vi "ErrorOut.vi"(1 "error in":errorcluster, 2 "DNL_NodeType":T1(ring)) -> (0 "error out":errorcluster)   [LabVIEW 2020]
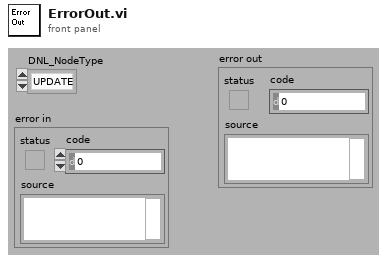
[diagram p1: front panel]
types:
  T1 = enum16{"UPDATE", "READ", "QUERY", "CREATE CHILD", "CREATE", "CONNECT", "DISCONNECT"}
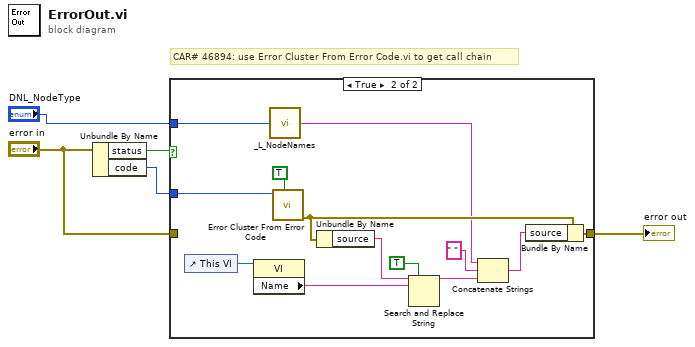
[diagram p0: block diagram]
diagram:
  # "CAR# 46894: use Error Cluster From Error Code.vi to get call chain"
  n1 = Unbundle By Name("error in") -> ("status"=w2:bool, "code"=w4:i32)
  n2 = case shown="True" w2 {
    tunnel: "DNL_NodeType" -> [_ w19]
    tunnel: w4 -> [_ w18]
    tunnel: [w6 w16] -> w3
    tunnel: "error in" -> [w6 _]
    frame False {
    }
    frame True {
      n3 = control-ref of="This VI"() -> (w15:refnum<vi>)
      n4 = property class="VI"(reference=w15) -> ("Name"=w12:string)  [unwired: 1 in, 2 out]
      n5 = call <vilib>:"_L_NodeNames.vi"("DNL_NodeType"=w19) -> ("DNL_NodeName"=w7:string)
      n6 = call <vilib>:"Error Cluster From Error Code.vi"("show call chain? (False)"=TRUE, "error code (0)"=w18) -> ("error out"=w14:errorcluster)  [unwired: 1 in, 6 out]
      n7 = Unbundle By Name(w14) -> ("source"=w13:string)
      n8 = Search and Replace String(replace all?=TRUE ("replace all? (F)"), input string=w13, search string=w12) -> (result string=w8:string)  [unwired: 2 in, 6 out]
      n9 = Concatenate Strings(w7, " " ("string"), w8) -> (w10:string)
      n10 = Bundle By Name(cluster=w14, "source"=w10) -> (w16:errorcluster)
    }
  }
  "error out" <- w3
